vi "5-2 shift register.vi"(0 "Numeric":i32=100) -> (1 "VALORE MIN":dbl format="%.8f", 2 "VALORE MAX":dbl format="%.8f")   [LabVIEW 2012]
doc: "M. Corti 2004"
panel:
  out "VALORI CASUALI":cluster{"number: 0 to 1":dbl, dbl, dbl}(graph)
  # "Utilizzare un ciclo FOR per calcolare in tempo reale il valore massimo ed il valore minimo di una serie di 100 numeri casuali. Rappresentare   i risultati con il valore generato in un grafico"
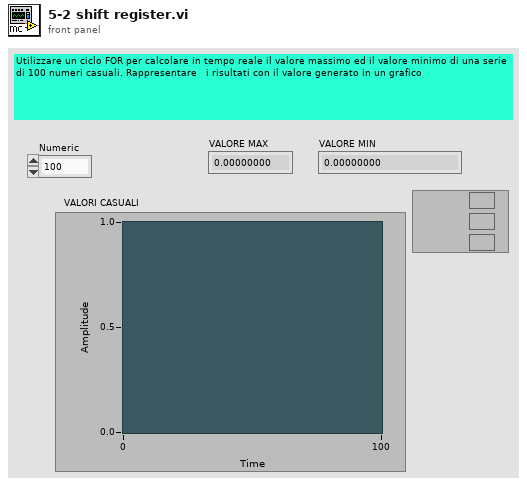
[diagram p1: front panel]
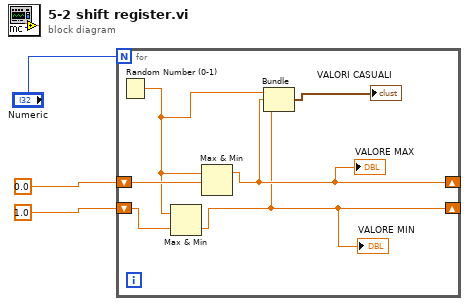
[diagram p0: block diagram]
diagram:
  n1 = for {
    N: "Numeric" -> [_]
    shift-right: [w5] -> _
    shift-left: 0.0 -> [w9]
    shift-right: [w4] -> _
    shift-left: 1.0 -> [w6]
    n2 = Random Number (0-1)() -> (number: 0 to 1=w8:dbl)
    n3 = Max & Min(x=w8, y=w6) -> (min(x,y)=w4:dbl)  [unwired: 1 out]
    "VALORE MIN" <- w4
    n4 = Max & Min(x=w8, y=w9) -> (max(x,y)=w5:dbl)  [unwired: 1 out]
    "VALORE MAX" <- w5
    n5 = Bundle("number: 0 to 1"=w8, w5, w4) -> (→"VALORI CASUALI":cluster{"number: 0 to 1":dbl, dbl, dbl})  [unwired: 1 in]
  }
